vi "Stop both app.vi"() -> ()   [LabVIEW 2018]
panel:
  out "STOP BOTH APP":bool
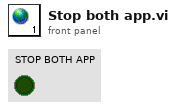
[diagram p1: front panel]
diagram:
